vi "SetVoltage.vi"(8 "error in (no error)":errorcluster, 10 "Voltage, V":dbl, 11 "SMU in":refnum<class "SMU.lvclass">) -> (0 "error out":errorcluster, 3 "SMU out":refnum<class "SMU.lvclass">)   [LabVIEW 2019, in "SMU.lvclass"]
uses:
  SMU.lvclass
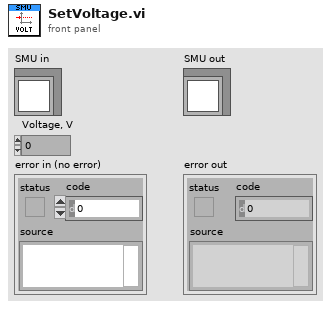
[diagram p1: front panel]
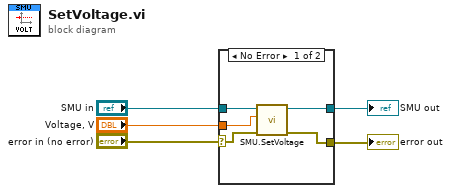
[diagram p0: block diagram]
diagram:
  n1 = case shown="No Error" "error in (no error)" {
    selector: "error in (no error)" -> [w9 w12]
    tunnel: [w6 w12] -> w4
    tunnel: [w7 w11] -> w2
    tunnel: "SMU in" -> [w10 w11]
    tunnel: "Voltage, V" -> [w8 _]
    frame No Error {
      n2 = call-dynamic "SMU.SetVoltage.vi"("error in (no error)"=w9, "Voltage, V"=w8, "SMU in"=w10) -> ("error out"=w6:errorcluster, "SMU out"=w7:refnum<class "SMU.lvclass">)  [unwired: 7 in]
    }
    frame Error {
    }
  }
  "error out" <- w4
  "SMU out" <- w2
